vi "Read Subpanels.vi"(8 "error in (no error)":errorcluster, 11 "Maui Manager in":refnum<class "Maui Manager.lvclass">) -> (0 "error out":errorcluster, 2 "Subpanels":refnum<class "SMO.lvclass">[](array[class]), 3 "Maui Manager out":refnum<class "Maui Manager.lvclass">)   [LabVIEW 2020, in "Maui Manager.lvclass"]
uses:
  Maui Manager.lvclass
  <vilib>/JKI/JKI SMO/SMO/SMO.lvclass
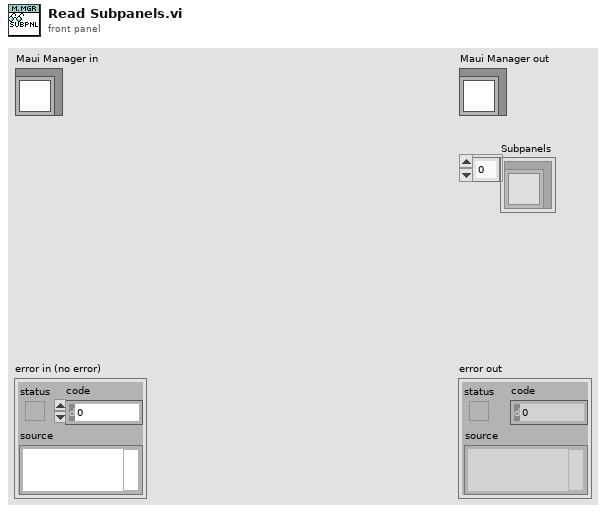
[diagram p1: front panel]
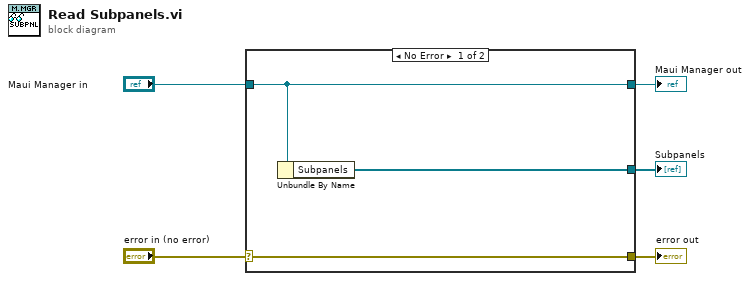
[diagram p0: block diagram]
diagram:
  n1 = case shown="No Error" "error in (no error)" {
    selector: "error in (no error)" -> [w8 w9]
    tunnel: [w8 w9] -> w4
    tunnel: [w7 w10] -> w2
    tunnel: "Maui Manager in" -> [w7 w10]
    tunnel: [w6 _] -> w1
    frame No Error {
      n2 = Unbundle By Name(w7) -> ("Subpanels"=w6:refnum<class "SMO.lvclass">[])
    }
    frame Error {
    }
  }
  "error out" <- w4
  "Maui Manager out" <- w2
  "Subpanels" <- w1
